vi "Set Initialization Data - First Level Worker.vi"(8 "error in":errorcluster, 11 "Head Worker in":refnum<class "Head Worker.lvclass">) -> (0 "error out":errorcluster, 3 "Head Worker out":refnum<class "Head Worker.lvclass">)   [LabVIEW 2017, in "Method 1.lvlib" / "Head Worker.lvclass"]
doc: "In this VI you can set the initialization data of a statically-linked subWorker."
uses:
  Head Worker.lvclass
  First Level Worker/Initialization Data.ctl
  First Level Worker/Response Cases.ctl
  <vilib>/addons/_Workers/Library/Case Label.ctl
  Head Worker.lvclass/Head Worker.ctl
  First Level Worker/First Level Worker.lvclass
  C:/Program Files (x86)/National Instruments/LabVIEW 2017/vi.lib/addons/_Workers/Library/Classes/Worker/Worker.lvclass
  <vilib>/addons/_Workers/Library/Workers.lvlib
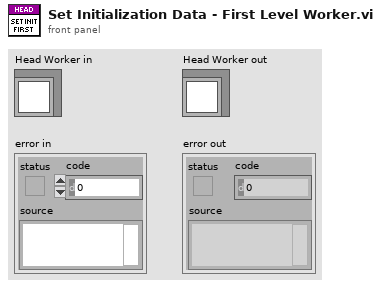
[diagram p1: front panel]
types:
  T1 = typedef "Method 1.lvlib/First Level Worker.lvclass/Initialization Data.ctl" = cluster{"Response Cases":T2}
  T2 = typedef "Method 1.lvlib/First Level Worker.lvclass/Response Cases.ctl" = cluster{"subWorker Error":T3}
  T3 = typedef "Workers.lvlib/Case Label.ctl" = string
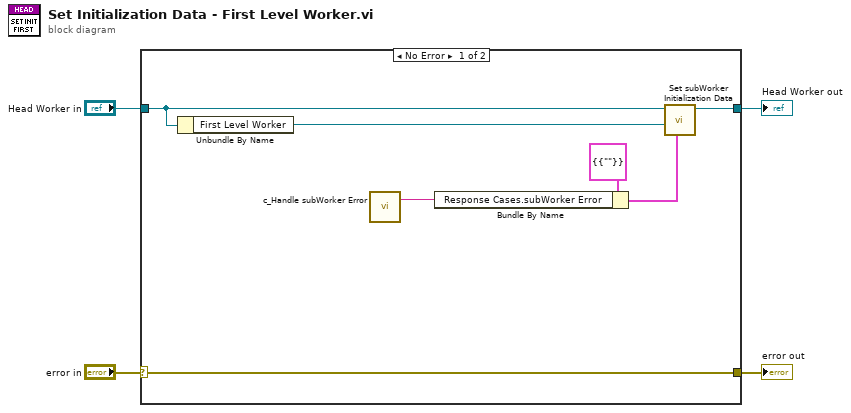
[diagram p0: block diagram]
diagram:
  n1 = case shown="No Error" "error in" {
    selector: "error in" -> [w11 w13]
    tunnel: [w11 w13] -> w3
    tunnel: [w9 w12] -> w2
    tunnel: "Head Worker in" -> [w8 w12]
    frame No Error {
      n2 = Unbundle By Name(w8) -> ("First Level Worker"=w10:refnum<class "First Level Worker.lvclass">)
      n3 = call "c_Handle subWorker Error.vi"() -> ("Case Label"=w5:T3)  [unwired: 1 in]
      n4 = Bundle By Name(cluster=T1 {"Response Cases"={"subWorker Error"=""}} ("Initialization Data"), "Response Cases.subWorker Error"=w5) -> (w6:T1)
      n5 = call-dynamic "Set subWorker Initialization Data.vi"("Initialization Data"=w6, "subWorker"=w10, "Worker"=w8) -> ("Worker out"=w9:refnum<class "Head Worker.lvclass">)  [unwired: 8 in]
    }
    frame Error {
    }
  }
  "error out" <- w3
  "Head Worker out" <- w2
